vi "Select Critical Point.vi"() -> ()   [LabVIEW 2010]
panel:
  out "Right Magnitude":dbl
  out "Left Magnitude":dbl
  out "Left Angle":dbl
  out "Right Angle":dbl
  in  "Y (mm)":dbl[](array[numeric])
  in  "X (mm)":dbl[](array[numeric])
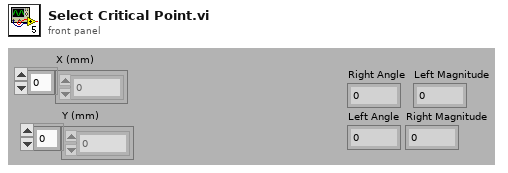
[diagram p1: front panel]
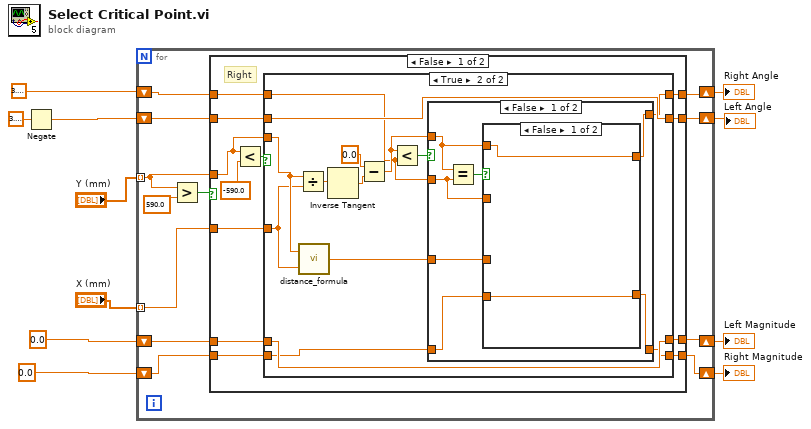
[diagram p0: block diagram]
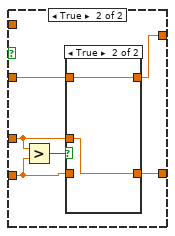
[diagram p3: hidden frame]
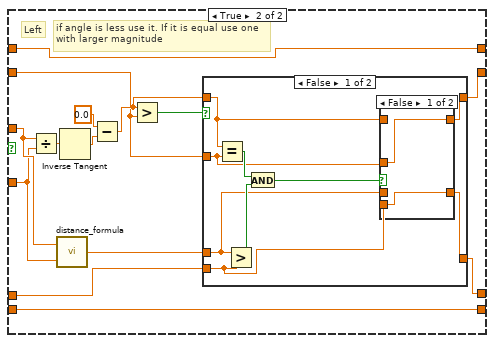
[diagram p6: hidden frame]
diagram:
  n1 = Negate(x=3.141592653589793) -> (-x=w8:dbl)
  n2 = for {
    tunnel: "Y (mm)" -> [w21] mode=indexing
    tunnel: "X (mm)" -> [w20] mode=indexing
    shift-right: [w18] -> w3
    shift-left: w8 -> [w19]
    shift-right: [w17] -> w2
    shift-left: 0.0 ("y") -> [w16]
    shift-right: [w14] -> w4
    shift-left: 3.141592653589793 -> [w15]
    shift-right: [w13] -> w1
    shift-left: 0.0 ("y") -> [w12]
    n3 = Greater?(x=w21, y=590.0) -> (0:w23:bool)
    n4 = case shown="False" w23 {
      tunnel: w21 -> [w24 w77]
      tunnel: w20 -> [w25 w75]
      tunnel: w19 -> [w33 w81]
      tunnel: [w32 w84] -> w18
      tunnel: [w30 w82] -> w17
      tunnel: w16 -> [w31 w80]
      tunnel: w15 -> [w29 w79]
      tunnel: [w28 w79] -> w14
      tunnel: [w26 w78] -> w13
      tunnel: w12 -> [w27 w78]
      frame False {
        # "Right"
        n5 = Less?(x=w24, y=-590.0) -> (x < y?=w35:bool)
        n6 = case shown="True" w35 {
          tunnel: w33 -> [w39 w46]
          tunnel: [w39 w46] -> w32
          tunnel: w31 -> [w38 w45]
          tunnel: [w38 w45] -> w30
          tunnel: w29 -> [w37 w44]
          tunnel: [w37 w41] -> w28
          tunnel: w27 -> [w36 w42]
          tunnel: [w36 w40] -> w26
          tunnel: w25 -> [_ w49]
          tunnel: w24 -> [_ w50]
          frame False {
          }
          frame True {
            n7 = Divide(x=w50, y=w49) -> (x/y=w51:dbl)
            n8 = call "distance_formula.vi"("X2 - X1"=w49, "Y2 - Y1"=w50) -> ("Distance"=w43:dbl)
            n9 = Inverse Tangent(1:w51) -> (0:w52:dbl)
            n10 = Subtract(x=0.0, y=w52) -> (x-y=w47:dbl)
            n11 = Less?(x=w47, y=w44) -> (x < y?=w48:bool)
            n12 = case shown="False" w48 {
              tunnel: w47 -> [w54 w74]
              tunnel: w44 -> [w57 _]
              tunnel: w43 -> [w59 _]
              tunnel: w42 -> [w58 w73]
              tunnel: [w56 w74] -> w41
              tunnel: [w55 w73] -> w40
              frame False {
                n13 = Equal?(x=w54, y=w57) -> (x = y?=w60:bool)
                n14 = case shown="False" w60 {
                  tunnel: w59 -> [_ w63]
                  tunnel: w58 -> [w61 w67]
                  tunnel: w57 -> [_ w66]
                  tunnel: [w62 w65] -> w56
                  tunnel: [w61 w64] -> w55
                  tunnel: w54 -> [w62 _]
                  frame False {
                  }
                  frame True {
                    n15 = Greater?(x=w63, y=w67) -> (0:w68:bool)
                    n16 = case shown="True" w68 {
                      tunnel: w67 -> [w69 _]
                      tunnel: w66 -> [w70 w71]
                      tunnel: [w70 w71] -> w65
                      tunnel: [w69 w72] -> w64
                      tunnel: w63 -> [_ w72]
                      frame False {
                      }
                      frame True {
                      }
                    }
                  }
                }
              }
              frame True {
              }
            }
          }
        }
      }
      frame True {
        # "if angle is less use it. If it is equal use one\nwith larger magnitude"
        # "Left"
        n17 = Divide(x=w77, y=w75) -> (x/y=w76:dbl)
        n18 = call "distance_formula.vi"("X2 - X1"=w75, "Y2 - Y1"=w77) -> ("Distance"=w83:dbl)
        n19 = Inverse Tangent(1:w76) -> (0:w88:dbl)
        n20 = Subtract(x=0.0, y=w88) -> (x-y=w85:dbl)
        n21 = Greater?(x=w85, y=w81) -> (0:w86:bool)
        n22 = case shown="False" w86 {
          tunnel: w85 -> [w92 w103]
          tunnel: [w91 w103] -> w84
          tunnel: w83 -> [w94 w102]
          tunnel: [w93 w102] -> w82
          tunnel: w81 -> [w90 _]
          tunnel: w80 -> [w89 _]
          frame False {
            n23 = Equal?(x=w92, y=w90) -> (x = y?=w96:bool)
            n24 = Greater?(x=w94, y=w89) -> (0:w97:bool)
            n25 = And(x=w96, y=w97) -> (x .and. y?=w95:bool)
            n26 = case shown="False" w95 {
              tunnel: w94 -> [_ w101]
              tunnel: [w98 w101] -> w93
              tunnel: w92 -> [_ w100]
              tunnel: [w99 w100] -> w91
              tunnel: w90 -> [w99 _]
              tunnel: w89 -> [w98 _]
              frame False {
              }
              frame True {
              }
            }
          }
          frame True {
          }
        }
      }
    }
  }
  "Right Angle" <- w4
  "Left Angle" <- w3
  "Left Magnitude" <- w2
  "Right Magnitude" <- w1
